vi "onUnsubscribe.vi"(6 "timeout (100ms)":i32=100, 8 "error in (no error)":errorcluster, 10 "UNSUBSCRIBE":refnum<class "UNSUBSCRIBE.lvclass">, 11 "Client in":refnum<class "Client.lvclass">) -> (0 "error out":errorcluster, 1 "Ack":bool, 2 "UNSUBACK":refnum<class "UNSUBACK.lvclass">, 3 "Client out":refnum<class "Client.lvclass">)   [LabVIEW 2013, in "MQTT Client.lvlib" / "Client.lvclass"]
uses:
  Client.lvclass
  <vilib>/LabVIEW Open Source Project/MQTT Control Packets/Control Packets/UNSUBSCRIBE/UNSUBSCRIBE.lvclass
  <vilib>/LabVIEW Open Source Project/MQTT Control Packets/Control Packets/UNSUBACK/UNSUBACK.lvclass
  <vilib>/LabVIEW Open Source Project/MQTT Control Packets/Control Packets/ControlPacket/ControlPacket.lvclass/ControlPacket.ctl
  MQTT_Base/Base Class/MQTT_Base.lvclass
  Client.lvclass/Client.ctl
  Session.Client/Session.Client.lvclass
  <vilib>/LabVIEW Open Source Project/MQTT Control Packets/Control Packets/ControlPacket/ControlPacket.lvclass
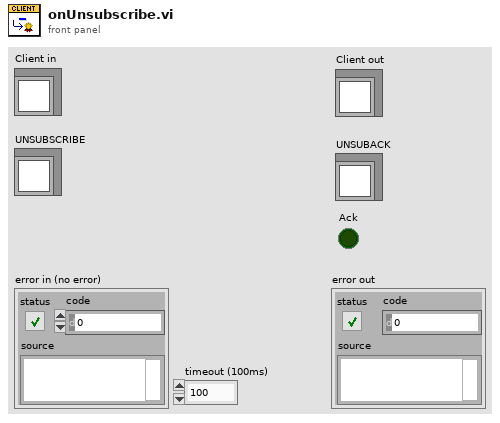
[diagram p1: front panel]
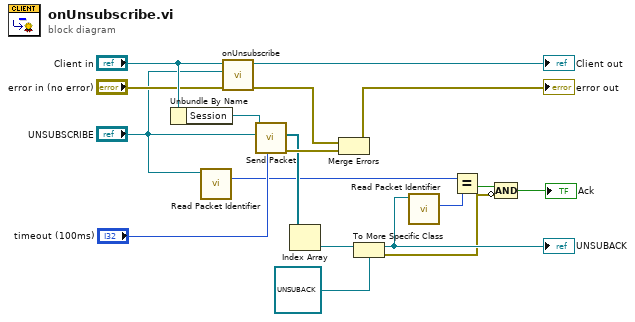
[diagram p0: block diagram]
diagram:
  n1 = Unbundle By Name("Client in") -> ("Session"=w18:refnum<class "Session.Client.lvclass">)
  n2 = call <vilib>:"Read Packet Identifier.vi"("ControlPacket in"="UNSUBSCRIBE") -> ("Packet Identifier"=w5:u16)  [unwired: 9 in, 1 out]
  n3 = call-parent "onUnsubscribe.vi"("error in (no error)"="error in (no error)", "UNSUBSCRIBE"="UNSUBSCRIBE", "MQTT_Base in"="Client in") -> ("error out"=w16:errorcluster, "MQTT_Base out"=→"Client out":refnum<class "Client.lvclass">)  [unwired: 5 in, 2 out]
  n4 = call "Send Packet.vi"("timeout (0ms : no ack)"="timeout (100ms)", "Packet"="UNSUBSCRIBE", "Session"=w18) -> ("error out"=w17:errorcluster, "Response"=w9:refnum<class "ControlPacket.lvclass">[])  [unwired: 5 in, 2 out]
  n5 = Index Array(array=w9) -> (element=w10:refnum<class "ControlPacket.lvclass">)  [unwired: 1 in]
  n6 = Merge Errors(w16, w17) -> (→"error out":errorcluster)
  n7 = To More Specific Class(target class=refnum<class "UNSUBACK.lvclass"> refnum ("UNSUBACK"), reference=w10) -> (specific class reference=w6:refnum<class "UNSUBACK.lvclass">, error out=w2:errorcluster)  [unwired: 1 in]
  "UNSUBACK" <- w6
  n8 = call <vilib>:"Read Packet Identifier.vi"("ControlPacket in"=w6) -> ("Packet Identifier"=w4:u16)  [unwired: 9 in, 1 out]
  n9 = Equal?(x=w5, y=w4) -> (x = y?=w3:bool)
  n10 = Compound Arithmetic op=AND(w3, invert w2) -> (→"Ack":bool)
